vi "Init HW.vi"(8 "error in (no error)":errorcluster, 9 "Clamp (Rake)":T3, 10 "Hardware Info":T1 {"Color Pane" items=["Blue", "Red", "Green", "Saturation", "Value", "Intensity", "Luminance", "Hue", ""]}, 11 "PWM Range":cluster{"High PW":dbl, "Low PW":dbl}) -> (0 "error out":errorcluster)   [LabVIEW 2020]
uses:
  Controls/HWchannels.ctl
  <vilib>/userdefined/High Color/IMAQdx.ctl
  Controls/HW States.ctl
panel:
  # "Channel"
  # "Frequency (Hz)"
  # "Force Sensor:"
  # "Servo:"
  # "LED:"
  # "N/A"
  # "Camera:"
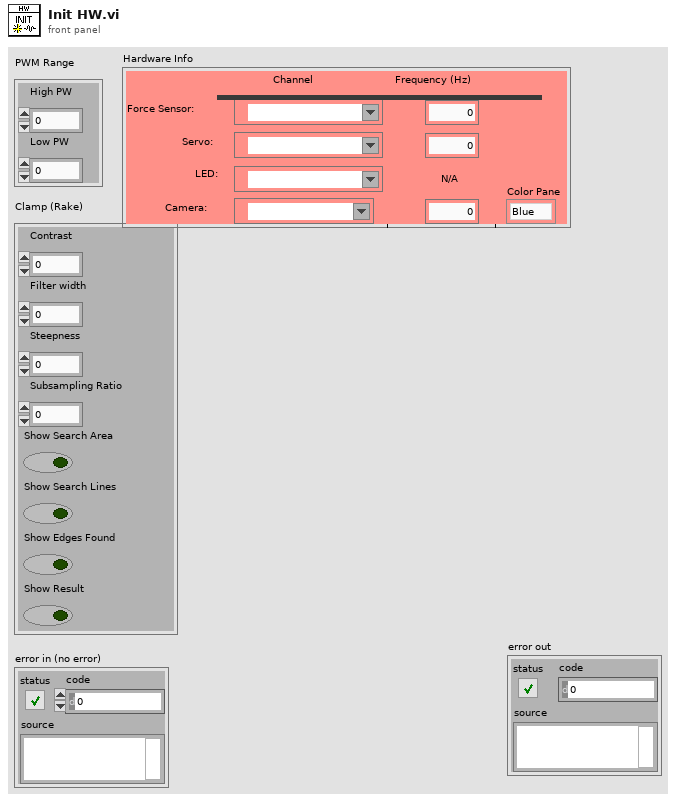
[diagram p1: front panel]
types:
  T1 = typedef "HWchannels.ctl" = cluster{"LED Channel":refnum<k21>, "Force Sensor Channel":tag, "Servo Channel":refnum<k21>, "Camera Selector":T2, "Camera Freq":dbl, "FS Freq":dbl, "Servo Freq":dbl, "Color Pane":i32}
  T2 = typedef "IMAQdx.ctl" = refnum<k21>
  T3 = cluster{"Contrast":i32, "Filter width":i32, "Steepness":i32, "Subsampling Ratio":u32, "Show Search Area":bool, "Show Search Lines":bool, "Show Edges Found":bool, "Show Result":bool}
  T4 = typedef "HW States.ctl" = enum16{"Initialize", "Input LED", "Input PWM", "Acquire Voltage", "Acquire Image", "Stop"}
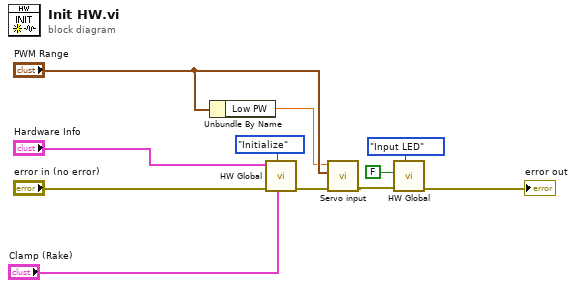
[diagram p0: block diagram]
diagram:
  n1 = Unbundle By Name("PWM Range") -> ("Low PW"=w10:dbl)
  n2 = call "HW Global.vi"("Clamp (Rake)"="Clamp (Rake)", "HW State"=HW_States."Initialize", "error in (no error)"="error in (no error)", "Hardware Info"="Hardware Info") -> ("error out"=w8:errorcluster)  [unwired: 4 in, 3 out]
  n3 = call "Servo input.vi"("error in (no error)"=w8, "PWM Range"="PWM Range", "Servo Input"=w10) -> ("error out"=w9:errorcluster)  [unwired: 8 in]
  n4 = call "HW Global.vi"("HW State"=HW_States."Input LED", "error in (no error)"=w9, "LED on?"=FALSE) -> ("error out"=→"error out":errorcluster)  [unwired: 5 in, 3 out]
